vi "XML Parser Tubes.vi"(8 "error in (no error)":errorcluster) -> (0 "error out":errorcluster, 3 "output array":string[](array[string]))   [LabVIEW 2023]
uses:
  <vilib>/xml/Close Reference(Node).vi
  <vilib>/xml/NI_XML.lvlib
  <resource>/objmgr/DOMUserDefRef.rc
panel:
  out "XML":string
  out "Parse Errors":string
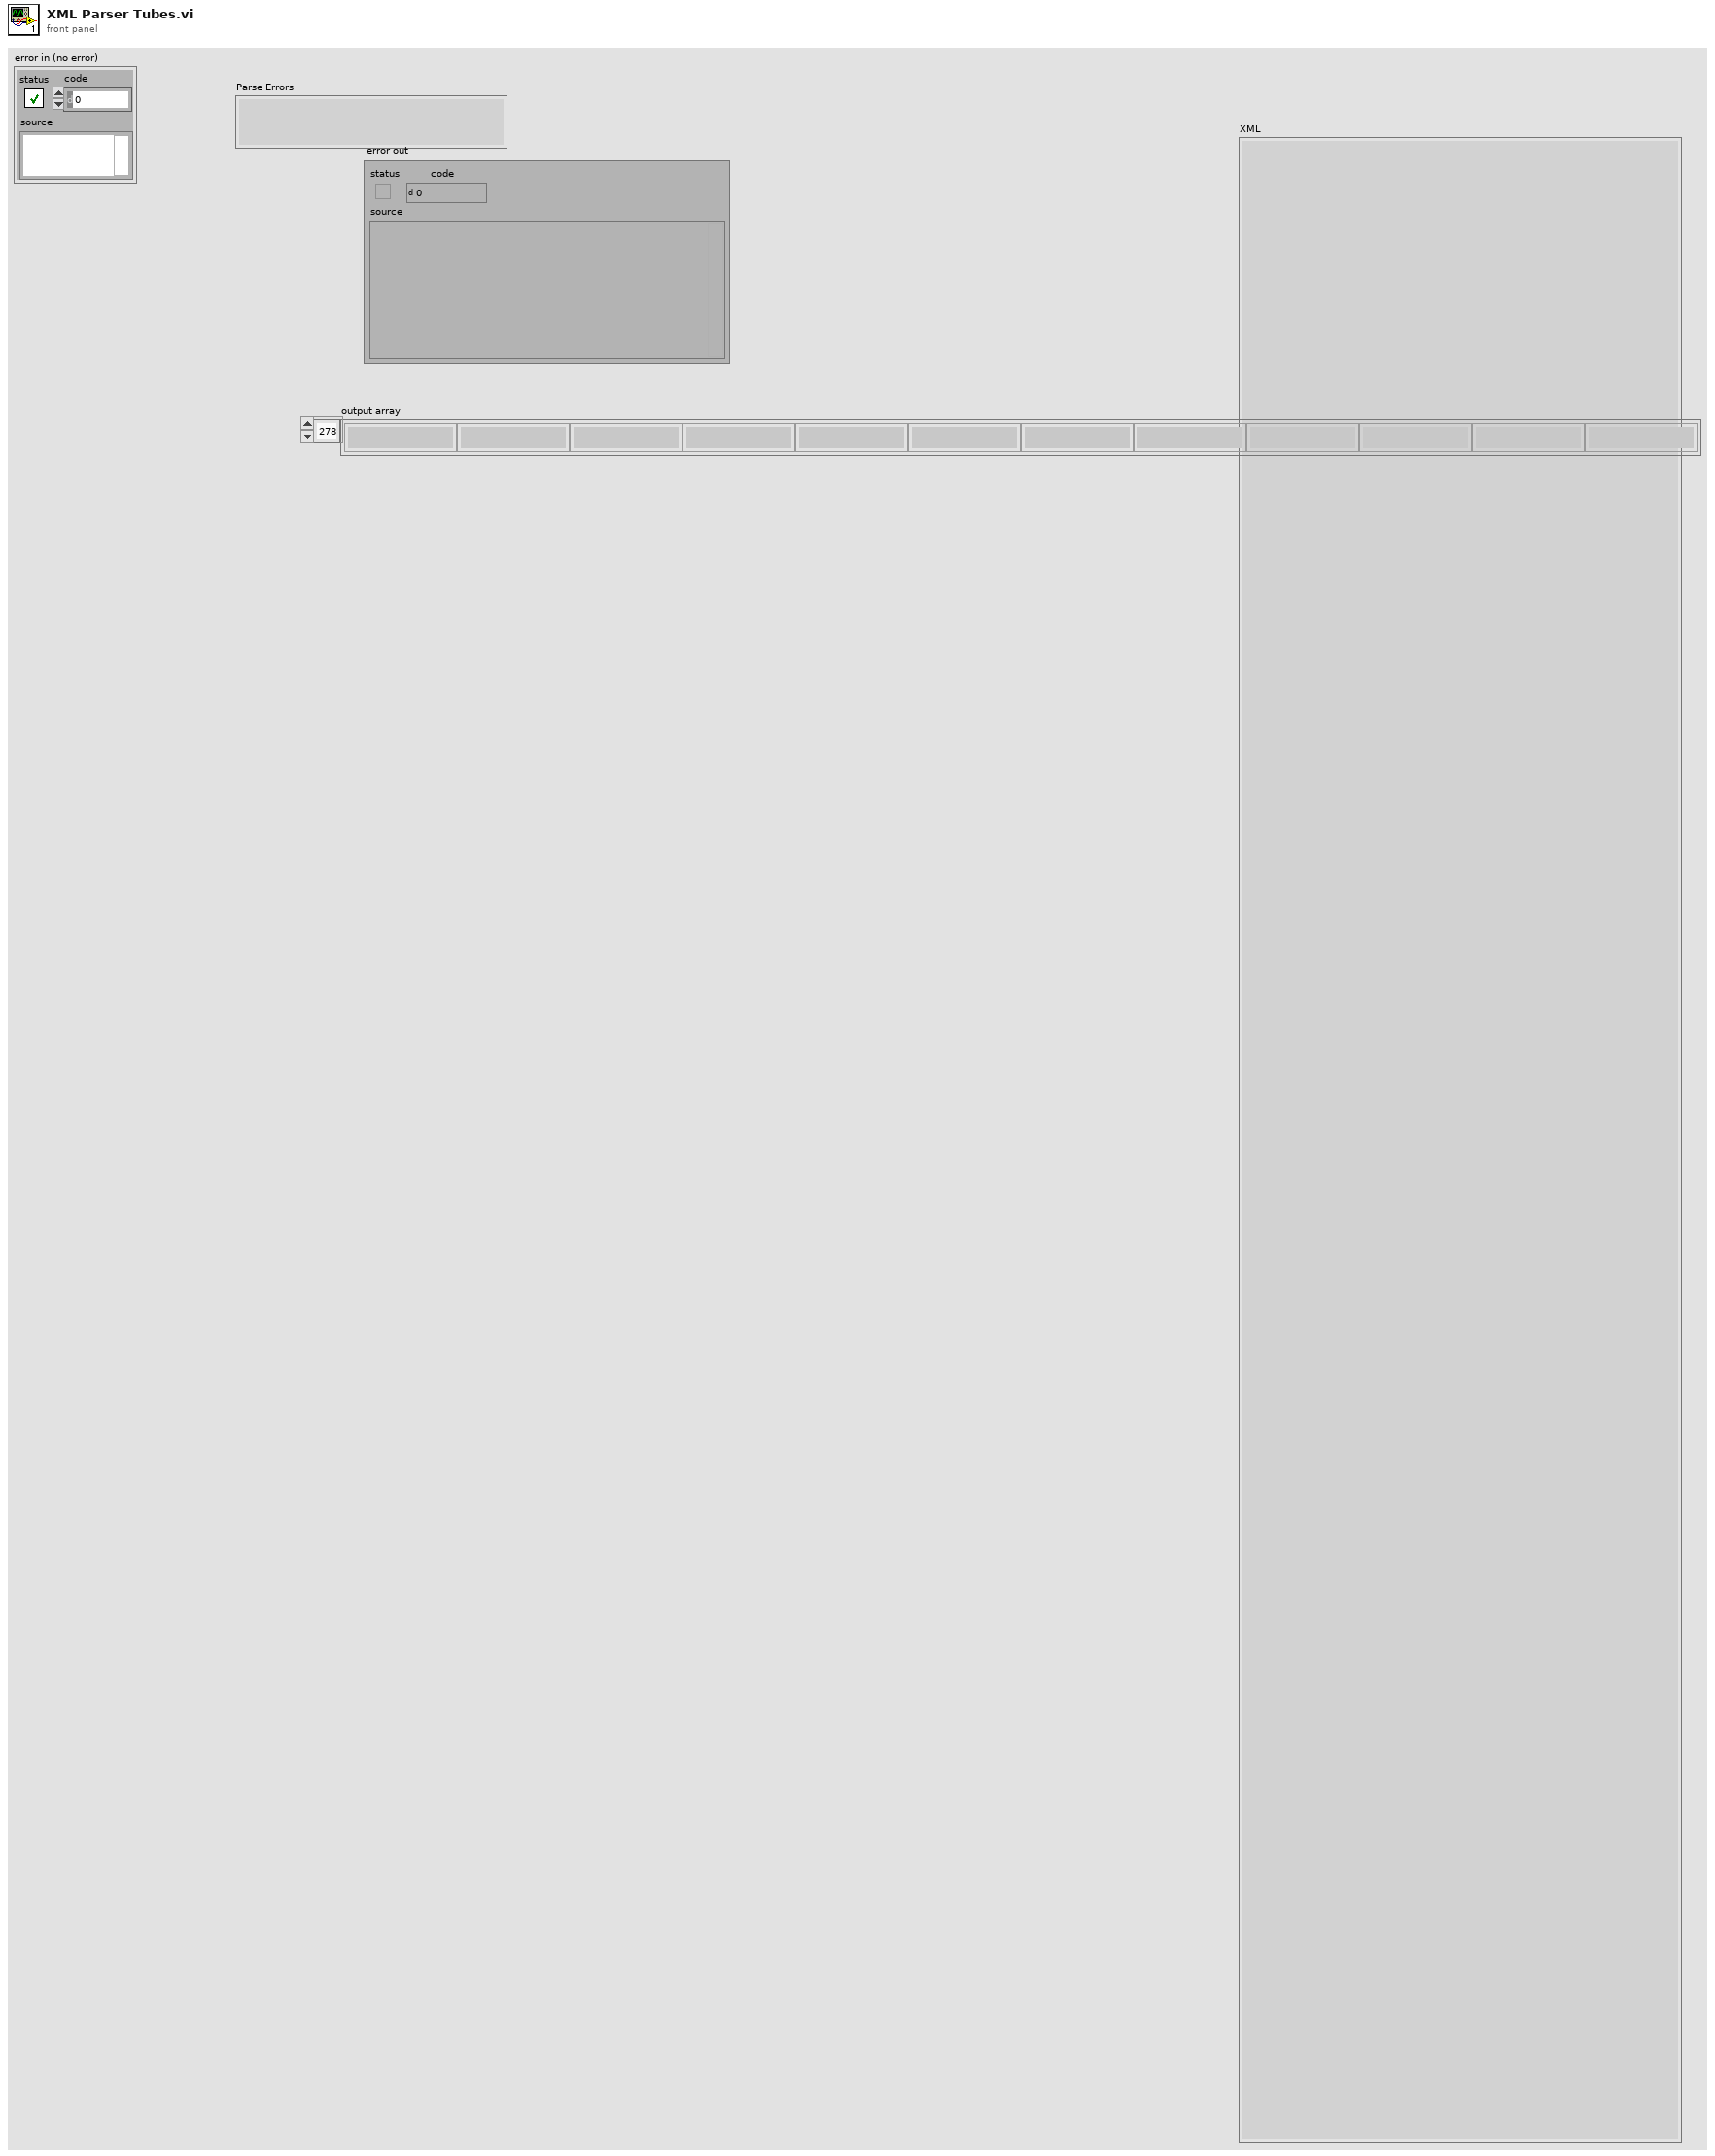
[diagram p1: front panel]
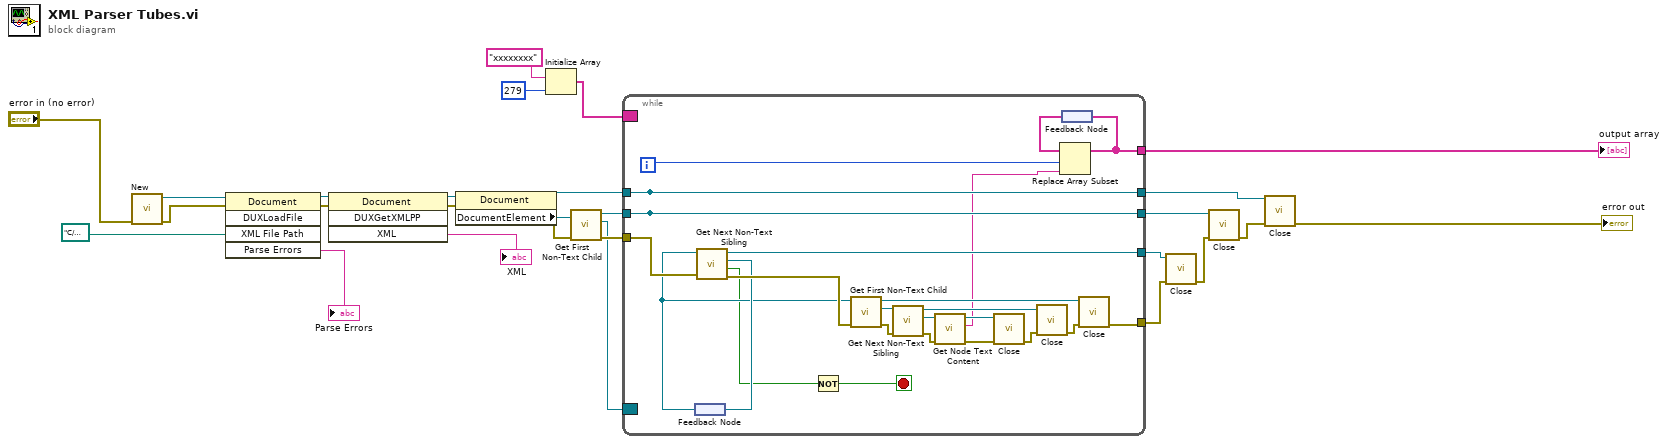
[diagram p0: block diagram]
diagram:
  n1 = call <vilib>:"New.vi"("error in (no error)"="error in (no error)") -> ("error out"=w26:errorcluster, "DOM document out"=w27:refnum<k20>)  [unwired: 7 in]
  n2 = invoke class="Document" method="DUXLoadFile"(reference=w27, error in=w26, "XML File Path"=path "C:/Users/Public/Documents/Grid2093/TUBES/tubetype.xsl" ("base path")) -> (reference out=w25:refnum<k20>, error out=w24:errorcluster, "Parse Errors"=→"Parse Errors":string)  [unwired: 2 in, 2 out]
  n3 = invoke class="Document" method="DUXGetXMLPP"(reference=w25, error in=w24) -> (reference out=w23:refnum<k20>, error out=w22:errorcluster, "XML"=→"XML":string)  [unwired: 2 in, 1 out]
  n4 = property class="Document"(reference=w23, error in=w22) -> (reference out=w16:refnum<k20>, error out=w17:errorcluster, "DocumentElement"=w18:refnum<k20>)
  n5 = Initialize Array("xxxxxxxx", 279 ("dimension size")) -> (w1:string[])
  n6 = call <vilib>:"Get First Non-Text Child.vi"("error in (no error)"=w17, "node in"=w18) -> ("error out"=w12:errorcluster, "child node"=w2:refnum<k20>, "node out"=w13:refnum<k20>)  [unwired: 6 in, 1 out]
  n7 = while {
    tunnel: w16 -> [w51]
    tunnel: w12 -> [w49]
    tunnel: w13 -> [w50]
    tunnel: [w51] -> _
    tunnel: [w50] -> _
    tunnel: [w51] -> w11
    tunnel: [w50] -> w10
    tunnel: [w34] -> w6
    tunnel: [w36] -> w5
    tunnel: [w35] -> w7
    border: w2 -> [_]
    border: w1 -> [_]
    i -> [w29]
    stop <- w28 stop-if-true
    n8 = feedback #1() -> (w32:refnum<k20>)
    n9 = call <vilib>:"Get Next Non-Text Sibling.vi"("error in (no error)"=w49, "node in"=w32) -> ("error out"=w38:errorcluster, "found sibling node?"=w30:bool, "sibling node"=w33:refnum<k20>, "node out"=w35:refnum<k20>)  [unwired: 6 in]
    n10 = feedback-in #1(w33) -> ()
    n11 = Not(x=w30) -> (.not. x?=w28:bool)
    n12 = call <vilib>:"Get First Non-Text Child.vi"("error in (no error)"=w38, "node in"=w32) -> ("error out"=w45:errorcluster, "child node"=w46:refnum<k20>, "node out"=w40:refnum<k20>)  [unwired: 6 in, 1 out]
    n13 = call <vilib>:"Get Next Non-Text Sibling.vi"("error in (no error)"=w45, "node in"=w46) -> ("error out"=w43:errorcluster, "sibling node"=w44:refnum<k20>, "node out"=w42:refnum<k20>)  [unwired: 6 in, 1 out]
    n14 = call <vilib>:"Get Node Text Content.vi"("error in (no error)"=w43, "node in"=w44) -> ("error out"=w48:errorcluster, "node text"=w31:string, "node out"=w47:refnum<k20>)  [unwired: 7 in]
    n15 = call-poly <vilib>:"Close.vi"("error in (no error)"=w48, "node"=w47) -> ("error out"=w41:errorcluster)  [unwired: 7 in]
    n16 = call-poly <vilib>:"Close.vi"("error in (no error)"=w41, "node"=w42) -> ("error out"=w39:errorcluster)  [unwired: 7 in]
    n17 = feedback #2() -> (w37:string[])
    n18 = Replace Array Subset(array=w37, new element=w31, index=w29) -> (w34:string[])
    n19 = feedback-in #2(w34) -> ()
    n20 = call-poly <vilib>:"Close.vi"("error in (no error)"=w39, "node"=w40) -> ("error out"=w36:errorcluster)  [unwired: 7 in]
  }
  "output array" <- w6
  n21 = call-poly <vilib>:"Close.vi"("error in (no error)"=w5, "node"=w7) -> ("error out"=w8:errorcluster)  [unwired: 7 in]
  n22 = call-poly <vilib>:"Close.vi"("error in (no error)"=w8, "node"=w10) -> ("error out"=w9:errorcluster)  [unwired: 7 in]
  n23 = call-poly <vilib>:"Close.vi"("error in (no error)"=w9, "node"=w11) -> ("error out"=→"error out":errorcluster)  [unwired: 7 in]
